vi "rsscope_core_global.vi"() -> ()   [LabVIEW 2014] (continued)
of the data signal in the USB 3.1 protocol.\n\nAvailable Repeated Capabilities:\nSerialBus: SB1, SB2, SB3, SB4\r\n\nRemote-control command(s):\nBUS<m>:USBThree:THRHigh"}, {"Level"=3, "Class Only"=FALSE, "Identifier"="RSSCOPE_ATTR_PROTOCOL_USB31_GEN1_SCRAMBLE_MODE", "Descriptive Name"="Protocol USB31 Gen1 Scramble Mode", "Data Type"=0, "Command"="BUS{SerialBus}:USBT:SCRM", "Access"=2, "Range Table"="RsScope_rngUSB31Gen1ScrambleMode", "Read Callback"="", "Write Callback"="", "Supported Models"="", "Instrument Options"="K61", "Flags"=0, "Help"="Selects if the data pattern is scrambled or unscambled.\n\nAvailable Repeated Capabilities:\nSerialBus: SB1, SB2, SB3, SB4\r\n\nRemote-control command(s):\nBUS<m>:USBThree:SCRMode"}, {"Level"=3, "Class Only"=FALSE, "Identifier"="RSSCOPE_ATTR_PROTOCOL_USB31_GEN1_TYPE", "Descriptive Name"="Protocol USB31 Gen1 Type", "Data Type"=0, "Command"="BUS{SerialBus}:USBT:TYPE", "Access"=2, "Range Table"="RsScope_rngProtocolUSB31Gen1Type", "Read Callback"="", "Write Callback"="", "Supported Models"="", "Instrument Options"="K61", "Flags"=0, "Help"="Selects the USB 3.1 protocol type.\n\nAvailable Repeated Capabilities:\nSerialBus: SB1, SB2, SB3, SB4\r\n\nRemote-control command(s):\nBUS<m>:USBThree:TYPE"}, {"Level"=3, "Class Only"=TRUE, "Identifier"="", "Descriptive Name"="Decoding Results", "Data Type"=0, "Command"="", "Access"=0, "Range Table"="", "Read Callback"="", "Write Callback"="", "Supported Models"="", "Instrument Options"="", "Flags"=0, "Help"="Returns the USB31 Generation1 decoding results."}, {"Level"=4, "Class Only"=FALSE, "Identifier"="RSSCOPE_ATTR_PROTOCOL_USB31_GEN1_FRAME_COUNT", "Descriptive Name"="Protocol USB31 Gen1 Frame Count", "Data Type"=0, "Command"="BUS{SerialBus}:USBT:RES:FCO?", "Access"=0, "Range Table"="", "Read Callback"="", "Write Callback"="", "Supported Models"="", "Instrument Options"="K61", "Flags"=0, "Help"="Returns the number of frames in the acquisition.\n\nAvailable Repeated Capabilities:\nSerialBus: SB1, SB2, SB3, SB4\r\n\nRemote-control command(s):\nBUS<m>:USBThree:RESult:FCOunt?"}, {"Level"=3, "Class Only"=TRUE, "Identifier"="", "Descriptive Name"="DSP", "Data Type"=0, "Command"="", "Access"=0, "Range Table"="", "Read Callback"="", "Write Callback"="", "Supported Models"="", "Instrument Options"="", "Flags"=0, "Help"="Here you can enable and define the equalization techniques used for the equalization at the reciever side of the signal."}, {"Level"=4, "Class Only"=FALSE, "Identifier"="RSSCOPE_ATTR_PROTOCOL_USB31_GEN1_TYPE_DSP_HIGH_SPEED_BITRATE", "Descriptive Name"="Protocol USB31 Gen1 Type DSP High Speed Bitrate", "Data Type"=1, "Command"="BUS{SerialBus}:USBT:BITR", "Access"=2, "Range Table"="RsScope_rngProtocolUSB31Gen1TypeDSPHighSpeedBitrate", "Read Callback"="", "Write Callback"="", "Supported Models"="", "Instrument Options"="K61", "Flags"=0, "Help"="Sets the bit rate.\n\nAvailable Repeated Capabilities:\nSerialBus: SB1, SB2, SB3, SB4\r\n\nRemote-control command(s):\nBUS<m>:USBThree:BITR"}, {"Level"=4, "Class Only"=TRUE, "Identifier"="", "Descriptive Name"="CTLE", "Data Type"=0, "Command"="", "Access"=0, "Range Table"="", "Read Callback"="", "Write Callback"="", "Supported Models"="", "Instrument Options"="", "Flags"=0, "Help"="Continuous time linear equalization (CTLE) is an equalization that can be used for improving the signal performance. It boosts the high frequency noise and the signal. Thus it helps reduce the inter-symbol interference (ISI) on the reciever side."}, {"Level"=5, "Class Only"=FALSE, "Identifier"="RSSCOPE_ATTR_PROTOCOL_USB31_GEN1_TYPE_DSP_CTLE_ENABLED", "Descriptive Name"="Protocol USB31 Gen1 Type DSP CTLE Enabled", "Data Type"=3, "Command"="BUS{SerialBus}:CTLE:ENBL", "Access"=2, "Range Table"="", "Read Callback"="", "Write Callback"="", "Supported Models"="", "Instrument Options"="K61", "Flags"=0, "Help"="Enables the continuous time linear equalization (CTLE) equalization.\n\nAvailable Repeated Capabilities:\nSerialBus: SB1, SB2, SB3, SB4\r\n\nRemote-control command(s):\nBUS<m>:CTLE:ENBLe"}, {"Level"=5, "Class Only"=FALSE, "Identifier"="RSSCOPE_ATTR_PROTOCOL_USB31_GEN1_TYPE_DSP_CTLE_ZERO_FREQUENCY", "Descriptive Name"="Protocol USB31 Gen1 Type DSP CTLE Zero Frequency", "Data Type"=1, "Command"="BUS{SerialBus}:CTLE:Z1FR", "Access"=2, "Range Table"="RsScope_rngProtocolUSB31Gen1TypeDSPCTLEFrequency", "Read Callback"="", "Write Callback"="", "Supported Models"="", "Instrument Options"="K61", "Flags"=0, "Help"="Sets the zero frequency for the transfer function of the CTLE algorithm.\n\nAvailable Repeated Capabilities:\nSerialBus: SB1, SB2, SB3, SB4\r\n\nRemote-control command(s):\nBUS<m>:CTLE:Z1FReq"}, {"Level"=5, "Class Only"=FALSE, "Identifier"="RSSCOPE_ATTR_PROTOCOL_USB31_GEN1_TYPE_DSP_CTLE_POLE_FREQUENCY_FP1", "Descriptive Name"="Protocol USB31 Gen1 Type DSP CTLE Pole Frequency FP1", "Data Type"=1, "Command"="BUS{SerialBus}:CTLE:P1FR", "Access"=2, "Range Table"="RsScope_rngProtocolUSB31Gen1TypeDSPCTLEFrequency", "Read Callback"="", "Write Callback"="", "Supported Models"="", "Instrument Options"="K61", "Flags"=0, "Help"="Sets the pole 1 frequency for the transfer function of the CTLE algorithm.\n\nAvailable Repeated Capabilities:\nSerialBus: SB1, SB2, SB3, SB4\r\n\nRemote-control command(s):\nBUS<m>:CTLE:P1FReq"}, {"Level"=5, "Class Only"=FALSE, "Identifier"="RSSCOPE_ATTR_PROTOCOL_USB31_GEN1_TYPE_DSP_CTLE_POLE_FREQUENCY_FP2", "Descriptive Name"="Protocol USB31 Gen1 Type DSP CTLE Pole Frequency FP2", "Data Type"=1, "Command"="BUS{SerialBus}:CTLE:P2FR", "Access"=2, "Range Table"="RsScope_rngProtocolUSB31Gen1TypeDSPCTLEFrequency", "Read Callback"="", "Write Callback"="", "Supported Models"="", "Instrument Options"="K61", "Flags"=0, "Help"="Sets the pole 2 frequency for the transfer function of the CTLE algorithm.\n\nAvailable Repeated Capabilities:\nSerialBus: SB1, SB2, SB3, SB4\r\n\nRemote-control command(s):\nBUS<m>:CTLE:P2FReq"}, {"Level"=5, "Class Only"=FALSE, "Identifier"="RSSCOPE_ATTR_PROTOCOL_USB31_GEN1_TYPE_DSP_CTLE_DC_GAIN", "Descriptive Name"="Protocol USB31 Gen1 Type DSP CTLE DC Gain", "Data Type"=1, "Command"="BUS{SerialBus}:CTLE:DCG", "Access"=2, "Range Table"="RsScope_rngProtocolUSB31Gen1TypeDSPCTLEDCGain", "Read Callback"="", "Write Callback"="", "Supported Models"="", "Instrument Options"="K61", "Flags"=0, "Help"="Sets the adjustable DC gain. This value can be chosen according to the channel loss characteristics. For low-loss channels, you can set a value close to 0 dB.\n\nAvailable Repeated Capabilities:\nSerialBus: SB1, SB2, SB3, SB4\r\n\nRemote-control command(s):\nBUS<m>:CTLE:DCGain"}, {"Level"=5, "Class Only"=FALSE, "Identifier"="RSSCOPE_ATTR_PROTOCOL_USB31_GEN1_TYPE_DSP_CTLE_CHANNEL_LENGTH", "Descriptive Name"="Protocol USB31 Gen1 Type DSP CTLE Channel Length", "Data Type"=0, "Command"="BUS{SerialBus}:USBT:PROT", "Access"=2, "Range Table"="RsScope_rngUSBDSPChannelLength", "Read Callback"="", "Write Callback"="", "Supported Models"="", "Instrument Options"="K61", "Flags"=0, "Help"="Selects the USB Super Speed channel length.\n\nAvailable Repeated Capabilities:\nSerialBus: SB1, SB2, SB3, SB4\r\n\nRemote-control command(s):\nBUS<m>:USBThree:PROTocol"}, {"Level"=4, "Class Only"=TRUE, "Identifier"="", "Descriptive Name"="DFE", "Data Type"=0, "Command"="", "Access"=0, "Range Table"="", "Read Callback"="", "Write Callback"="", "Supported Models"="", "Instrument Options"="", "Flags"=0, "Help"="Defines the settings of the decision feedback equalization (DFE). DFE correction is needed when the channel is distosrted."}, {"Level"=5, "Class Only"=FALSE, "Identifier"="RSSCOPE_ATTR_PROTOCOL_USB31_GEN1_TYPE_DSP_DFE_ENABLED", "Descriptive Name"="Protocol USB31 Gen1 Type DSP DFE Enabled", "Data Type"=3, "Command"="BUS{SerialBus}:USBT:DFE:ENBL", "Access"=2, "Range Table"="", "Read Callback"="", "Write Callback"="", "Supported Models"="", "Instrument Options"="K61", "Flags"=0, "Help"="Enables the use of the decision feedback equalization for USB 3.1.\n\nAvailable Repeated Capabilities:\nSerialBus: SB1, SB2, SB3, SB4\r\n\nRemote-control command(s):\nBUS<m>:USBThree:DFE:ENBLe"}, {"Level"=5, "Class Only"=FALSE, "Identifier"="RSSCOPE_ATTR_PROTOCOL_USB31_GEN1_TYPE_DSP_DFE_ESTIMATE_COEFFICIENTS_ENABLED", "Descriptive Name"="Protocol USB31 Gen1 Type DSP DFE Estimate Coefficients Enabled", "Data Type"=3, "Command"="BUS{SerialBus}:USBT:DFE:ESTC", "Access"=2, "Range Table"="", "Read Callback"="", "Write Callback"="", "Supported Models"="", "Instrument Options"="K61", "Flags"=0, "Help"="Enables the use of estimate coefficients for the decision feedback equalization.\n\nAvailable Repeated Capabilities:\nSerialBus: SB1, SB2, SB3, SB4\r\n\nRemote-control command(s):\nBUS<m>:USBThree:DFE:ESTCoeff"}, {"Level"=5, "Class Only"=FALSE, "Identifier"="RSSCOPE_ATTR_PROTOCOL_USB31_GEN1_TYPE_DSP_DFE_COEFFICIENT", "Descriptive Name"="Protocol USB31 Gen1 Type DSP DFE Coefficient", "Data Type"=1, "Command"="BUS{SerialBus}:USBT:DFE:COEF", "Access"=2, "Range Table"="RsScope_rngDSPDFECoefficient", "Read Callback"="", "Write Callback"="", "Supported Models"="", "Instrument Options"="K61", "Flags"=0, "Help"="Sets the value of the coefficient for the DFE.\n\nAvailable Repeated Capabilities:\nSerialBus: SB1, SB2, SB3, SB4\r\n\nRemote-control command(s):\nBUS<m>:USBThree:DFE:COEFficient"}, {"Level"=5, "Class Only"=FALSE, "Identifier"="RSSCOPE_ATTR_PROTOCOL_USB31_GEN1_TYPE_DSP_DFE_NUMBER_OF_TAPS", "Descriptive Name"="Protocol USB31 Gen1 Type DSP DFE Number Of Taps", "Data Type"=0, "Command"="BUS{SerialBus}:USBT:DFE:TCON", "Access"=2, "Range Table"="RsScope_rngDSPDFENumberOfTaps", "Read Callback"="", "Write Callback"="", "Supported Models"="", "Instrument Options"="K61", "Flags"=0, "Help"="Sets a number of taps for the decision feedback filter.\n\nAvailable Repeated Capabilities:\nSerialBus: SB1, SB2, SB3, SB4\r\n\nRemote-control command(s):\nBUS<m>:USBThree:DFE:TCONt"}, {"Level"=2, "Class Only"=TRUE, "Identifier"="", "Descriptive Name"="USB PD", "Data Type"=0, "Command"="", "Access"=0, "Range Table"="", "Read Callback"="", "Write Callback"="", "Supported Models"="", "Instrument Options"="", "Flags"=0, "Help"="R&S RTO-K63 is a firmware option that enables the R&S RTO to analyze Universal Serial Bus Power Delivery (USBPD) signals."}, {"Level"=3, "Class Only"=FALSE, "Identifier"="RSSCOPE_ATTR_PROTOCOL_USB_PD_DATA_SOURCE", "Descriptive Name"="Protocol USB PD Data Source", "Data Type"=0, "Command"="BUS{SerialBus}:USBP:SOUR", "Access"=2, "Range Table"="rsscope_rngProtocolWaveformSource", "Read Callback"="", "Write Callback"="", "Supported Models"="", "Instrument Options"="", "Flags"=0, "Help"="Selects the source for the data signal in the USBPD protocol.\n\nAvailable Repeated Capabilities:\nSerialBus: SB1, SB2, SB3, SB4\r\n\nRemote-control command(s):\nBUS<m>:USBPd:SOURce"}, {"Level"=3, "Class Only"=FALSE, "Identifier"="RSSCOPE_ATTR_PROTOCOL_USB_PD_DATA_THRESHOLD", "Descriptive Name"="Protocol USB PD Data Threshold", "Data Type"=1, "Command"="BUS{SerialBus}:USBP:THR", "Access"=2, "Range Table"="RsScope_rngUSBPDThreshold", "Read Callback"="", "Write Callback"="", "Supported Models"="", "Instrument Options"="K63", "Flags"=0, "Help"="Sets the threshold value of the data.\n\nAvailable Repeated Capabilities:\nSerialBus: SB1, SB2, SB3, SB4\r\n\nRemote-control command(s):\nBUS<m>:USBPd:THReshold"}, {"Level"=3, "Class Only"=FALSE, "Identifier"="RSSCOPE_ATTR_PROTOCOL_USB_PD_DATA_HYSTERESIS", "Descriptive Name"="Protocol USB PD Data Hysteresis", "Data Type"=1, "Command"="BUS{SerialBus}:USBP:HYST", "Access"=2, "Range Table"="RsScope_rngUSBPDDataHysteresis", "Read Callback"="", "Write Callback"="", "Supported Models"="", "Instrument Options"="K63", "Flags"=0, "Help"="Sets a value for the hysteresis of the data.\n\nAvailable Repeated Capabilities:\nSerialBus: SB1, SB2, SB3, SB4\r\n\nRemote-control command(s):\nBUS<m>:USBPd:HYSTeresis"}, {"Level"=3, "Class Only"=FALSE, "Identifier"="RSSCOPE_ATTR_PROTOCOL_USB_PD_THRESHOLD_VRD15", "Descriptive Name"="Protocol USB PD Threshold VRD15", "Data Type"=1, "Command"="BUS{SerialBus}:USBP:THRB", "Access"=2, "Range Table"="RsScope_rngUSBPDThreshold", "Read Callback"="", "Write Callback"="", "Supported Models"="", "Instrument Options"="K63", "Flags"=0, "Help"="Sets the bottom threshold (for the low current ) for the current advertisment mode.\n\nAvailable Repeated Capabilities:\nSerialBus: SB1, SB2, SB3, SB4\r\n\nRemote-control command(s):\nBUS<m>:USBPd:THRBottom"}, {"Level"=3, "Class Only"=FALSE, "Identifier"="RSSCOPE_ATTR_PROTOCOL_USB_PD_THRESHOLD_VRD_USB", "Descriptive Name"="Protocol USB PD Threshold VRD USB", "Data Type"=1, "Command"="BUS{SerialBus}:USBP:THRM", "Access"=2, "Range Table"="RsScope_rngUSBPDThreshold", "Read Callback"="", "Write Callback"="", "Supported Models"="", "Instrument Options"="K63", "Flags"=0, "Help"="Sets the middle threshold (at default USB Type-C currnet) for the current advertisment mode.\n\nAvailable Repeated Capabilities:\nSerialBus: SB1, SB2, SB3, SB4\r\n\nRemote-control command(s):\nBUS<m>:USBPd:THRMid"}, {"Level"=3, "Class Only"=FALSE, "Identifier"="RSSCOPE_ATTR_PROTOCOL_USB_PD_THRESHOLD_VRA", "Descriptive Name"="Protocol USB PD Threshold VRA", "Data Type"=1, "Command"="BUS{SerialBus}:USBP:THRT", "Access"=2, "Range Table"="RsScope_rngUSBPDThreshold", "Read Callback"="", "Write Callback"="", "Supported Models"="", "Instrument Options"="K63", "Flags"=0, "Help"="Sets the top threshold (at USB Type-C currnet of 1.5 A ) for the current advertisment mode\n\nAvailable Repeated Capabilities:\nSerialBus: SB1, SB2, SB3, SB4\r\n\nRemote-control command(s):\nBUS<m>:USBPd:THRTop"}, {"Level"=3, "Class Only"=FALSE, "Identifier"="RSSCOPE_ATTR_PROTOCOL_USB_PD_SHOW_DECODE_DETAIL", "Descriptive Name"="Protocol USB PD Show Decode Detail", "Data Type"=3, "Command"="BUS{SerialBus}:USBP:DET", "Access"=2, "Range Table"="", "Read Callback"="", "Write Callback"="", "Supported Models"="", "Instrument Options"="K63", "Flags"=0, "Help"="If enabled, the data words are broken down into subframes. If not enabled the data words are displayed as 32-bit data words.\n\nAvailable Repeated Capabilities:\nSerialBus: SB1, SB2, SB3, SB4\r\n\nRemote-control command(s):\nBUS<m>:USBPd:DETail"}, {"Level"=3, "Class Only"=TRUE, "Identifier"="", "Descriptive Name"="Decoding Results", "Data Type"=0, "Command"="", "Access"=0, "Range Table"="", "Read Callback"="", "Write Callback"="", "Supported Models"="", "Instrument Options"="", "Flags"=0, "Help"="Returns the USB PD decoding results."}, {"Level"=4, "Class Only"=FALSE, "Identifier"="RSSCOPE_ATTR_PROTOCOL_USB_PD_FRAME_COUNT", "Descriptive Name"="Protocol USB PD Frame Count", "Data Type"=0, "Command"="BUS{SerialBus}:USBP:RES:FCO?", "Access"=0, "Range Table"="", "Read Callback"="", "Write Callback"="", "Supported Models"="", "Instrument Options"="K63", "Flags"=0, "Help"="Returns the number of frames in the acquisition.\n\nAvailable Repeated Capabilities:\nSerialBus: SB1, SB2, SB3, SB4\r\n\nRemote-control command(s):\nBUS<m>:USBPd:RESult:FCOunt?"}, {"Level"=2, "Class Only"=TRUE, "Identifier"="", "Descriptive Name"="Custom Manchester NRZ", "Data Type"=0, "Command"="", "Access"=0, "Range Table"="", "Read Callback"="", "Write Callback"="", "Supported Models"="", "Instrument Options"="", "Flags"=0, "Help"="R&S RTO-K50 is a firmware option that enables the R&S RTO to analyze customizable serial bus signals encoded by the following coding standards: Manchester, Manchester II, NRZ Clocked, NRZ Unclocked."}, {"Level"=3, "Class Only"=FALSE, "Identifier"="RSSCOPE_ATTR_PROTOCOL_MANCHESTER_NRZ_CODING_STANDARD", "Descriptive Name"="Protocol Manchester NRZ Coding Standard", "Data Type"=0, "Command"="BUS{SerialBus}:CMSB:COD", "Access"=2, "Range Table"="RsScope_rngManchesterNRZCodingStandard", "Read Callback"="", "Write Callback"="", "Supported Models"="", "Instrument Options"="K50", "Flags"=0, "Help"="Selects the custom serial bus coding standard.\n\nAvailable Repeated Capabilities:\nSerialBus: SB1, SB2, SB3, SB4\r\n\nRemote-control command(s):\nBUS<m>:CMSB:CODing"}, {"Level"=3, "Class Only"=FALSE, "Identifier"="RSSCOPE_ATTR_PROTOCOL_MANCHESTER_NRZ_BITRATE_ENABLED", "Descriptive Name"="Protocol Manchester NRZ Bitrate Enabled", "Data Type"=3, "Command"="BUS{SerialBus}:CMSB:BITR:ENAB", "Access"=2, "Range Table"="", "Read Callback"="", "Write Callback"="", "Supported Models"="", "Instrument Options"="K50", "Flags"=0, "Help"="Enables the bit rate settings (must always be enabled for the coding standard &apos;NRZ Unclocked&apos;, and also for triggering on signals in any coding standard).\n\nAvailable Repeated Capabilities:\nSerialBus: SB1, SB2, SB3, SB4\r\n\nRemote-control command(s):\nBUS<m>:CMSB:BITRate:ENABle"}, {"Level"=3, "Class Only"=FALSE, "Identifier"="RSSCOPE_ATTR_PROTOCOL_MANCHESTER_NRZ_BITRATE", "Descriptive Name"="Protocol Manchester NRZ Bitrate", "Data Type"=0, "Command"="BUS{SerialBus}:CMSB:BITR:VAL", "Access"=2, "Range Table"="RsScope_rngManchesterNRZBitrate", "Read Callback"="", "Write Callback"="", "Supported Models"="", "Instrument Options"="K50", "Flags"=0, "Help"="Sets the transmission speed setting for the custom serial bus data signal.\n\nAvailable Repeated Capabilities:\nSerialBus: SB1, SB2, SB3, SB4\r\n\nRemote-control command(s):\nBUS<m>:CMSB:BITRate:VALue"}, {"Level"=3, "Class Only"=FALSE, "Identifier"="RSSCOPE_ATTR_PROTOCOL_MANCHESTER_NRZ_GAP_TIME_ENABLED", "Descriptive Name"="Protocol Manchester NRZ Gap Time Enabled", "Data Type"=3, "Command"="BUS{SerialBus}:CMSB:GAPT:ENAB", "Access"=2, "Range Table"="", "Read Callback"="", "Write Callback"="", "Supported Models"="", "Instrument Options"="K50", "Flags"=0, "Help"="Enables the gap time settings (must always be enabled for the coding standard &apos;NRZ Unclocked&apos;, and also for triggering on signals in any coding standard).\n\nAvailable Repeated Capabilities:\nSerialBus: SB1, SB2, SB3, SB4\r\n\nRemote-control command(s):\nBUS<m>:CMSB:GAPTime:ENABle"}, {"Level"=3, "Class Only"=FALSE, "Identifier"="RSSCOPE_ATTR_PROTOCOL_MANCHESTER_NRZ_GAP_TIME", "Descriptive Name"="Protocol Manchester NRZ Gap Time", "Data Type"=1, "Command"="BUS{SerialBus}:CMSB:GAPT:VAL", "Access"=2, "Range Table"="RsScope_rngManchesterNRZGapTime", "Read Callback"="", "Write Callback"="", "Supported Models"="", "Instrument Options"="K50", "Flags"=0, "Help"="Sets a minimum gap time for synchronization.\n\nAvailable Repeated Capabilities:\nSerialBus: SB1, SB2, SB3, SB4\r\n\nRemote-control command(s):\nBUS<m>:CMSB:GAPTime:VALue"}, {"Level"=3, "Class Only"=TRUE, "Identifier"="", "Descriptive Name"="Manchester", "Data Type"=0, "Command"="", "Access"=0, "Range Table"="", "Read Callback"="", "Write Callback"="", "Supported Models"="", "Instrument Options"="", "Flags"=0, "Help"="Configures manchester coding standard."}, {"Level"=4, "Class Only"=FALSE, "Identifier"="RSSCOPE_ATTR_PROTOCOL_MANCHESTER_DATA_SOURCE", "Descriptive Name"="Protocol Manchester Data Source", "Data Type"=0, "Command"="BUS{SerialBus}:CMSB:MANC:DATA", "Access"=2, "Range Table"="rsscope_rngProtocolWaveformSource", "Read Callback"="", "Write Callback"="", "Supported Models"="", "Instrument Options"="K50", "Flags"=0, "Help"="Selects the source channel for the data signal. For triggering on a serial bus, analog channels C1 - C4  are required. Otherwise, if no serial bus trigger has been selected, permitted source selections include the mathematical channels and the reference channels.\n\nAvailable Repeated Capabilities:\nSerialBus: SB1, SB2, SB3, SB4\r\n\nRemote-control command(s):\nBUS<m>:CMSB:MANChester:DATA"}, {"Level"=4, "Class Only"=FALSE, "Identifier"="RSSCOPE_ATTR_PROTOCOL_MANCHESTER_POLARITY", "Descriptive Name"="Protocol Manchester Polarity", "Data Type"=0, "Command"="BUS{SerialBus}:CMSB:MANC:POL", "Access"=2, "Range Table"="rsscope_rngPolarityNormalInverted", "Read Callback"="", "Write Callback"="", "Supported Models"="", "Instrument Options"="K50", "Flags"=0, "Help"="Selects the polarity of the custom serial bus data signal in Manchester coding standards.\n\nAvailable Repeated Capabilities:\nSerialBus: SB1, SB2, SB3, SB4\r\n\nRemote-control command(s):\nBUS<m>:CMSB:MANChester:POLarity"}, {"Level"=4, "Class Only"=FALSE, "Identifier"="RSSCOPE_ATTR_PROTOCOL_MANCHESTER_CLOCK_PHASE", "Descriptive Name"="Protocol Manchester Clock Phase", "Data Type"=0, "Command"="BUS{SerialBus}:CMSB:MANC:CPH", "Access"=2, "Range Table"="RsScope_rngClockPhase", "Read Callback"="", "Write Callback"="", "Supported Models"="", "Instrument Options"="K50", "Flags"=0, "Help"="Selects the phase of the custom serial bus clock signal for the &apos;Manchester&apos; coding standards.\n\nAvailable Repeated Capabilities:\nSerialBus: SB1, SB2, SB3, SB4\r\n\nRemote-control command(s):\nBUS<m>:CMSB:MANChester:CPHase"}, {"Level"=4, "Class Only"=FALSE, "Identifier"="RSSCOPE_ATTR_PROTOCOL_MANCHESTER_THRESHOLD_LOW", "Descriptive Name"="Protocol Manchester Threshold Low", "Data Type"=1, "Command"="BUS{SerialBus}:CMSB:MANC:THR:LOW", "Access"=2, "Range Table"="RsScope_rngNRZThreshold", "Read Callback"="", "Write Callback"="", "Supported Models"="", "Instrument Options"="K50", "Flags"=0, "Help"="Sets the lower threshold for data signal digitization in Manchester coding standards.\n\nAvailable Repeated Capabilities:\nSerialBus: SB1, SB2, SB3, SB4\r\n\nRemote-control command(s):\nBUS<m>:CMSB:MANChester:THReshold:LOW"}, {"Level"=4, "Class Only"=FALSE, "Identifier"="RSSCOPE_ATTR_PROTOCOL_MANCHESTER_THRESHOLD_HIGH", "Descriptive Name"="Protocol Manchester Threshold High", "Data Type"=1, "Command"="BUS{SerialBus}:CMSB:MANC:THR:HIGH", "Access"=2, "Range Table"="RsScope_rngProtocolManchesterThresholdHigh", "Read Callback"="", "Write Callback"="", "Supported Models"="", "Instrument Options"="K50", "Flags"=0, "Help"="Sets the upper threshold for data signal digitization in Manchester coding standards.\n\nAvailable Repeated Capabilities:\nSerialBus: SB1, SB2, SB3, SB4\r\n\nRemote-control command(s):\nBUS<m>:CMSB:MANChester:THReshold:HIGH"}, {"Level"=4, "Class Only"=FALSE, "Identifier"="RSSCOPE_ATTR_PROTOCOL_MANCHESTER_THRESHOLD_PRESET", "Descriptive Name"="Protocol Manchester Threshold Preset", "Data Type"=0, "Command"="BUS{SerialBus}:CMSB:MANC:THR:PRES", "Access"=2, "Range Table"="RsScope_rngManchesterNRZThresholdPreset", "Read Callback"="", "Write Callback"="", "Supported Models"="", "Instrument Options"="K50", "Flags"=0, "Help"="Sets the Manchester thresholds to predefined or individually definable voltage levels.\n\nAvailable Repeated Capabilities:\nSerialBus: SB1, SB2, SB3, SB4\r\n\nRemote-control command(s):\nBUS<m>:CMSB:MANChester:THReshold:PRESet"}, {"Level"=4, "Class Only"=FALSE, "Identifier"="RSSCOPE_ATTR_PROTOCOL_MANCHESTER_THRESHOLD_COUPLING", "Descriptive Name"="Protocol Manchester Threshold Coupling", "Data Type"=3, "Command"="BUS{SerialBus}:CMSB:MANC:THR:COUP", "Access"=2, "Range Table"="", "Read Callback"="", "Write Callback"="", "Supported Models"="", "Instrument Options"="K50", "Flags"=0, "Help"="Couples the upper and lower threshold values for the Manchester and Manchester II coding standards. The values are coupled to voltages with the same magnitude but opposite sign (positive for the upper threshold and negative for the lower threshold).\n\nAvailable Repeated Capabilities:\nSerialBus: SB1, SB2, SB3, SB4\r\n\nRemote-control command(s):\nBUS<m>:CMSB:MANChester:THReshold:COUPling"}, {"Level"=3, "Class Only"=TRUE, "Identifier"="", "Descriptive Name"="NRZ", "Data Type"=0, "Command"="", "Access"=0, "Range Table"="", "Read Callback"="", "Write Callback"="", "Supported Models"="", "Instrument Options"="", "Flags"=0, "Help"="Configures NRZ coding standard."}, {"Level"=4, "Class Only"=FALSE, "Identifier"="RSSCOPE_ATTR_PROTOCOL_NRZ_DATA_SOURCE", "Descriptive Name"="Protocol NRZ Data Source", "Data Type"=0, "Command"="BUS{SerialBus}:CMSB:NRZ:DATA", "Access"=2, "Range Table"="rsscope_rngProtocolWaveformSource", "Read Callback"="", "Write Callback"="", "Supported Models"="", "Instrument Options"="K50", "Flags"=0, "Help"="Selects the source channel for the data signal in NRZ coding standards. For triggering on the serial bus when the NRZ clocked coding standard is selected, analog or digital channel sources are required. For triggering on the serial bus when the NRZ unclocked coding standard is selected, analog channel sources are required. Otherwise, if no serial bus trigger has been selected, permitted source selections include the mathematical channels and the reference channels.\n\nAvailable Repeated Capabilities:\nSerialBus: SB1, SB2, SB3, SB4\r\n\nRemote-control command(s):\nBUS<m>:CMSB:NRZ:DATA"}, {"Level"=4, "Class Only"=FALSE, "Identifier"="RSSCOPE_ATTR_PROTOCOL_NRZ_ENABLE_SOURCE", "Descriptive Name"="Protocol NRZ Enable Source", "Data Type"=0, "Command"="BUS{SerialBus}:CMSB:NRZ:ENBL", "Access"=2, "Range Table"="rsscope_rngProtocolWaveformSource", "Read Callback"="", "Write Callback"="", "Supported Models"="", "Instrument Options"="K50", "Flags"=0, "Help"="Selects the input source for the custom serial bus enable signal.\nIf an input is chosen, signals will be only decoded while this channel is in the enabled state. This allows you to mark a time when the signal on the selected source is active and when not.\n\nAvailable Repeated Capabilities:\nSerialBus: SB1, SB2, SB3, SB4\r\n\nRemote-control command(s):\nBUS<m>:CMSB:NRZ:ENBLe"}, {"Level"=4, "Class Only"=FALSE, "Identifier"="RSSCOPE_ATTR_PROTOCOL_NRZ_CLOCK_SOURCE", "Descriptive Name"="Protocol NRZ Clock Source", "Data Type"=0, "Command"="BUS{SerialBus}:CMSB:NRZ:CLCK", "Access"=2, "Range Table"="rsscope_rngProtocolWaveformSource", "Read Callback"="", "Write Callback"="", "Supported Models"="", "Instrument Options"="K50", "Flags"=0, "Help"="Selects the source channel for the clock signal in the NRZ Clocked coding standard. For triggering on the serial bus when the NRZ clocked coding standard is selected, analog or digital channel sources are required. Otherwise, if no serial bus trigger has been selected, permitted source selections include the mathematical channels and the reference channels.\n\nAvailable Repeated Capabilities:\nSerialBus: SB1, SB2, SB3, SB4\r\n\nRemote-control command(s):\nBUS<m>:CMSB:NRZ:CLCK"}, {"Level"=4, "Class Only"=FALSE, "Identifier"="RSSCOPE_ATTR_PROTOCOL_NRZ_POLARITY", "Descriptive Name"="Protocol NRZ Polarity", "Data Type"=0, "Command"="BUS{SerialBus}:CMSB:NRZ:POL", "Access"=2, "Range Table"="rsscope_rngActivePolarity", "Read Callback"="", "Write Callback"="", "Supported Models"="", "Instrument Options"="K50", "Flags"=0, "Help"="Selects the polarity of the custom serial bus data signal in NRZ coding standards.\n\nAvailable Repeated Capabilities:\nSerialBus: SB1, SB2, SB3, SB4\r\n\nRemote-control command(s):\nBUS<m>:CMSB:NRZ:POLarity"}, {"Level"=4, "Class Only"=FALSE, "Identifier"="RSSCOPE_ATTR_PROTOCOL_NRZ_ENA_POLARITY", "Descriptive Name"="Protocol NRZ ENA Polarity", "Data Type"=0, "Command"="BUS{SerialBus}:CMSB:NRZ:ENAP", "Access"=2, "Range Table"="RsScope_rngNRZPolarityData", "Read Callback"="", "Write Callback"="", "Supported Models"="", "Instrument Options"="K50", "Flags"=0, "Help"="Sets whether the transmitted enable signal is active when the voltage is below the threshold (ENALow) or higher than it (ENAHIgh).\n\nAvailable Repeated Capabilities:\nSerialBus: SB1, SB2, SB3, SB4\r\n\nRemote-control command(s):\nBUS<m>:CMSB:NRZ:ENAPolarity"}, {"Level"=4, "Class Only"=FALSE, "Identifier"="RSSCOPE_ATTR_PROTOCOL_NRZ_IDLE_POLARITY_UNCLOCKED", "Descriptive Name"="Protocol NRZ Idle Polarity Unclocked", "Data Type"=0, "Command"="BUS{SerialBus}:CMSB:NRZ:IDLP", "Access"=2, "Range Table"="rsscope_rngProtocolPolarity", "Read Callback"="", "Write Callback"="", "Supported Models"="", "Instrument Options"="K50", "Flags"=0, "Help"="Selects the idle polarity of the custom serial bus data signal (only available for the coding standard &apos;NRZ Unclocked&apos;).\n\nAvailable Repeated Capabilities:\nSerialBus: SB1, SB2, SB3, SB4\r\n\nRemote-control command(s):\nBUS<m>:CMSB:NRZ:IDLPolarity"}, {"Level"=4, "Class Only"=FALSE, "Identifier"="RSSCOPE_ATTR_PROTOCOL_NRZ_IDLE_POLARITY_CLOCKED", "Descriptive Name"="Protocol NRZ Idle Polarity Clocked", "Data Type"=0, "Command"="BUS{SerialBus}:CMSB:NRZ:CPOL", "Access"=2, "Range Table"="rsscope_rngProtocolPolarity", "Read Callback"="", "Write Callback"="", "Supported Models"="", "Instrument Options"="K50", "Flags"=0, "Help"="Selects the custom serial bus clock signal polarity for the coding standard NRZ Clocked.\n\nAvailable Repeated Capabilities:\nSerialBus: SB1, SB2, SB3, SB4\r\n\nRemote-control command(s):\nBUS<m>:CMSB:NRZ:CPOLarity"}, {"Level"=4, "Class Only"=FALSE, "Identifier"="RSSCOPE_ATTR_PROTOCOL_NRZ_CLOCK_PHASE", "Descriptive Name"="Protocol NRZ Clock Phase", "Data Type"=0, "Command"="BUS{SerialBus}:CMSB:NRZ:CPH", "Access"=2, "Range Table"="RsScope_rngNRZClockPhase", "Read Callback"="", "Write Callback"="", "Supported Models"="", "Instrument Options"="K50", "Flags"=0, "Help"="Selects the phase of the custom serial bus clock signal for the NRZ coding standards.\n\nAvailable Repeated Capabilities:\nSerialBus: SB1, SB2, SB3, SB4\r\n\nRemote-control command(s):\nBUS<m>:CMSB:NRZ:CPHase"}, {"Level"=4, "Class Only"=FALSE, "Identifier"="RSSCOPE_ATTR_PROTOCOL_NRZ_THRESHOLD_CLOCK", "Descriptive Name"="Protocol NRZ Threshold Clock", "Data Type"=1, "Command"="BUS{SerialBus}:CMSB:NRZ:THR:CLCK", "Access"=2, "Range Table"="RsScope_rngNRZThreshold", "Read Callback"="", "Write Callback"="", "Supported Models"="", "Instrument Options"="K50", "Flags"=0, "Help"="Sets the threshold for the clock signal digitization in the NRZ Clocked coding standard.\n\nAvailable Repeated Capabilities:\nSerialBus: SB1, SB2, SB3, SB4\r\n\nRemote-control command(s):\nBUS<m>:CMSB:NRZ:THReshold:CLCK"}, {"Level"=4, "Class Only"=FALSE, "Identifier"="RSSCOPE_ATTR_PROTOCOL_NRZ_THRESHOLD_DATA", "Descriptive Name"="Protocol NRZ Threshold Data", "Data Type"=1, "Command"="BUS{SerialBus}:CMSB:NRZ:THR:DATA", "Access"=2, "Range Table"="RsScope_rngNRZThreshold", "Read Callback"="", "Write Callback"="", "Supported Models"="", "Instrument Options"="K50", "Flags"=0, "Help"="Sets the threshold for the data signal digitization in NRZ coding standards.\n\nAvailable Repeated Capabilities:\nSerialBus: SB1, SB2, SB3, SB4\r\n\nRemote-control command(s):\nBUS<m>:CMSB:NRZ:THReshold:DATA"}, {"Level"=4, "Class Only"=FALSE, "Identifier"="RSSCOPE_ATTR_PROTOCOL_NRZ_THRESHOLD_PRESET", "Descriptive Name"="Protocol NRZ Threshold Preset", "Data Type"=0, "Command"="BUS{SerialBus}:CMSB:NRZ:THR:PRES", "Access"=2, "Range Table"="RsScope_rngManchesterNRZThresholdPreset", "Read Callback"="", "Write Callback"="", "Supported Models"="", "Instrument Options"="K50", "Flags"=0, "Help"="Sets the NRZ thresholds to predefined or individually definable voltage levels.\n\nAvailable Repeated Capabilities:\nSerialBus: SB1, SB2, SB3, SB4\r\n\nRemote-control command(s):\nBUS<m>:CMSB:NRZ:THReshold:PRESet"}, {"Level"=4, "Class Only"=FALSE, "Identifier"="RSSCOPE_ATTR_PROTOCOL_NRZ_THRESHOLD_COUPLING", "Descriptive Name"="Protocol NRZ Threshold Coupling", "Data Type"=3, "Command"="BUS{SerialBus}:CMSB:NRZ:THR:COUP", "Access"=2, "Range Table"="", "Read Callback"="", "Write Callback"="", "Supported Models"="", "Instrument Options"="K50", "Flags"=0, "Help"="Couples the clock and data threshold values for the NRZ Clocked coding standard. The values are coupled to the same number.\n\nAvailable Repeated Capabilities:\nSerialBus: SB1, SB2, SB3, SB4\r\n\nRemote-control command(s):\nBUS<m>:CMSB:NRZ:THReshold:COUPling"}, {"Level"=4, "Class Only"=FALSE, "Identifier"="RSSCOPE_ATTR_PROTOCOL_NRZ_THRESHOLD_VALUE", "Descriptive Name"="Protocol NRZ Threshold Value", "Data Type"=1, "Command"="BUS{SerialBus}:CMSB:NRZ:THR:ENBL", "Access"=2, "Range Table"="RsScope_rngNRZThresholdEnabled", "Read Callback"="", "Write Callback"="", "Supported Models"="", "Instrument Options"="K50", "Flags"=0, "Help"="Sets the threshold for the enable signal digitization in NRZ coding standards.\n\nAvailable Repeated Capabilities:\nSerialBus: SB1, SB2, SB3, SB4\r\n\nRemote-control command(s):\nBUS<m>:CMSB:NRZ:THReshold:ENBLe"}, {"Level"=4, "Class Only"=FALSE, "Identifier"="RSSCOPE_ATTR_PROTOCOL_NRZ_HYSTERESIS_CLOCK", "Descriptive Name"="Protocol NRZ Hysteresis Clock", "Data Type"=1, "Command"="BUS{SerialBus}:CMSB:NRZ:HYST:CLCK", "Access"=2, "Range Table"="RsScope_rngNRZHysteresis", "Read Callback"="", "Write Callback"="", "Supported Models"="", "Instrument Options"="K50", "Flags"=0, "Help"="Sets the hysteresis size on the clock channel.\n\nAvailable Repeated Capabilities:\nSerialBus: SB1, SB2, SB3, SB4\r\n\nRemote-control command(s):\nBUS<m>:CMSB:NRZ:HYSTeresis:CLCK"}, {"Level"=4, "Class Only"=FALSE, "Identifier"="RSSCOPE_ATTR_PROTOCOL_NRZ_HYSTERESIS_DATA", "Descriptive Name"="Protocol NRZ Hysteresis Data", "Data Type"=1, "Command"="BUS{SerialBus}:CMSB:NRZ:HYST:DATA", "Access"=2, "Range Table"="RsScope_rngNRZHysteresis", "Read Callback"="", "Write Callback"="", "Supported Models"="", "Instrument Options"="K50", "Flags"=0, "Help"="Sets the hysteresis size on the data line channel.\n\nAvailable Repeated Capabilities:\nSerialBus: SB1, SB2, SB3, SB4\r\n\nRemote-control command(s):\nBUS<m>:CMSB:NRZ:HYSTeresis:DATA"}, {"Level"=4, "Class Only"=FALSE, "Identifier"="RSSCOPE_ATTR_PROTOCOL_NRZ_HYSTERESIS_ENABLE_VALUE", "Descriptive Name"="Protocol NRZ Hysteresis Enable Value", "Data Type"=1, "Command"="BUS{SerialBus}:CMSB:NRZ:HYST:ENBL", "Access"=2, "Range Table"="RsScope_rngNRZHysteresis", "Read Callback"="", "Write Callback"="", "Supported Models"="", "Instrument Options"="K50", "Flags"=0, "Help"="Sets the hysteresis size on the enable line channel.\n\nAvailable Repeated Capabilities:\nSerialBus: SB1, SB2, SB3, SB4\r\n\nRemote-control command(s):\nBUS<m>:CMSB:NRZ:HYSTeresis:ENBLe"}, {"Level"=3, "Class Only"=TRUE, "Identifier"="", "Descriptive Name"="Frame Format", "Data Type"=0, "Command"="", "Access"=0, "Range Table"="", "Read Callback"="", "Write Callback"="", "Supported Models"="", "Instrument Options"="", "Flags"=0, "Help"="Configures frame format."}, {"Level"=4, "Class Only"=FALSE, "Identifier"="RSSCOPE_ATTR_PROTOCOL_MANCHESTER_NRZ_SELECTED_FRAME", "Descriptive Name"="Protocol Manchester NRZ Selected Frame", "Data Type"=0, "Command"="", "Access"=2, "Range Table"="", "Read Callback"="", "Write Callback"="", "Supported Models"="", "Instrument Options"="", "Flags"=0, "Help"="Sets selector repeated capability Frame.\n\nAvailable Repeated Capabilities:\nNone\n\nRemote-control command(s):\n"}, {"Level"=4, "Class Only"=FALSE, "Identifier"="RSSCOPE_ATTR_PROTOCOL_MANCHESTER_NRZ_FRAME_COUNT", "Descriptive Name"="Protocol Manchester NRZ Frame Count", "Data Type"=0, "Command"="BUS{SerialBus}:CMSB:FCO?", "Access"=0, "Range Table"="", "Read Callback"="", "Write Callback"="", "Supported Models"="", "Instrument Options"="K50", "Flags"=0, "Help"="Returns the frame count.\n\nAvailable Repeated Capabilities:\nSerialBus: SB1, SB2, SB3, SB4\r\n\nRemote-control command(s):\nBUS<m>:CMSB:FCOunt?"}, {"Level"=4, "Class Only"=FALSE, "Identifier"="RSSCOPE_ATTR_PROTOCOL_MANCHESTER_NRZ_FRAME_TYPE", "Descriptive Name"="Protocol Manchester NRZ Frame Type", "Data Type"=2, "Command"="BUS{SerialBus}:CMSB:FRAM<Frame>:TYPE", "Access"=2, "Range Table"="", "Read Callback"="rsscope_FormatManchesterNRZFrameRepCapString_ReadCallback.vi", "Write Callback"="rsscope_FormatManchesterNRZFrameRepCapString_WriteCallback.vi", "Supported Models"="", "Instrument Options"="K50", "Flags"=0, "Help"="Enables the user to set a string to describe the frame type, typically according to the applicable protocol standard specifications. (For example, MDIO (Option R&S RTO-K55) defines the frames READ, WRITE, ADDRESS, etc.)\n\nAvailable Repeated Capabilities:\nSerialBus: SB1, SB2, SB3, SB4\r\n\nRemote-control command(s):\nBUS<m>:CMSB:FRAMe<n>:TYPE"}, {"Level"=4, "Class Only"=FALSE, "Identifier"="RSSCOPE_ATTR_PROTOCOL_MANCHESTER_NRZ_ADD_FRAME", "Descriptive Name"="Protocol Manchester NRZ Add Frame", "Data Type"=4, "Command"="BUS{SerialBus}:CMSB:ADDF", "Access"=1, "Range Table"="", "Read Callback"="", "Write Callback"="", "Supported Models"="", "Instrument Options"="K50", "Flags"=0, "Help"="Creates an empty frame format description and adds it to the end of the frame description list.\n\nAvailable Repeated Capabilities:\nSerialBus: SB1, SB2, SB3, SB4\r\n\nRemote-control command(s):\nBUS<m>:CMSB:ADDFrame"}, {"Level"=4, "Class Only"=FALSE, "Identifier"="RSSCOPE_ATTR_PROTOCOL_MANCHESTER_NRZ_FRAME_CLEAR", "Descriptive Name"="Protocol Manchester NRZ Frame Clear", "Data Type"=4, "Command"="BUS{SerialBus}:CMSB:CLR", "Access"=1, "Range Table"="", "Read Callback"="", "Write Callback"="", "Supported Models"="", "Instrument Options"="K50", "Flags"=0, "Help"="Erases all cells and frames that have been created for a specific custom protocol.\n\nAvailable Repeated Capabilities:\nSerialBus: SB1, SB2, SB3, SB4\r\n\nRemote-control command(s):\nBUS<m>:CMSB:CLR"}, {"Level"=4, "Class Only"=FALSE, "Identifier"="RSSCOPE_ATTR_PROTOCOL_MANCHESTER_NRZ_FRAME_OPEN_DESCRIPTION", "Descriptive Name"="Protocol Manchester NRZ Frame Open Description", "Data Type"=2, "Command"="BUS{SerialBus}:CMSB:LOAD", "Access"=1, "Range Table"="", "Read Callback"="", "Write Callback"="", "Supported Models"="", "Instrument Options"="K50", "Flags"=0, "Help"="Opens an existing frame description file in xml format. The default path is \\\\Public\\Documents\\Rohde-Schwarz\\RTx\\SaveXML\n\nAvailable Repeated Capabilities:\nSerialBus: SB1, SB2, SB3, SB4\r\n\nRemote-control command(s):\nBUS<m>:CMSB:LOAD"}, {"Level"=4, "Class Only"=FALSE, "Identifier"="RSSCOPE_ATTR_PROTOCOL_MANCHESTER_NRZ_FRAME_SAVE_DESCRIPTION", "Descriptive Name"="Protocol Manchester NRZ Frame Save Description", "Data Type"=2, "Command"="BUS{SerialBus}:CMSB:SAVE", "Access"=1, "Range Table"="", "Read Callback"="", "Write Callback"="", "Supported Models"="", "Instrument Options"="K50", "Flags"=0, "Help"="Saves a created frame description into an xml file (&apos;Save As...&apos;). The default path is \\\\Public\\Documents\\Rohde-Schwarz\\RTx\\SaveXML\n\nAvailable Repeated Capabilities:\nSerialBus: SB1, SB2, SB3, SB4\r\n\nRemote-control command(s):\nBUS<m>:CMSB:SAVE"}, {"Level"=4, "Class Only"=FALSE, "Identifier"="RSSCOPE_ATTR_PROTOCOL_MANCHESTER_NRZ_EXPORT_FRAMES_AS_RAW_BITS", "Descriptive Name"="Protocol Manchester NRZ Export Frames As Raw Bits", "Data Type"=4, "Command"="BUS{SerialBus}:CMSB:EXRB", "Access"=1, "Range Table"="", "Read Callback"="", "Write Callback"="", "Supported Models"="", "Instrument Options"="K50", "Flags"=0, "Help"="Exports the decoded frames as raw bits.\n\nAvailable Repeated Capabilities:\nSerialBus: SB1, SB2, SB3, SB4\r\n\nRemote-control command(s):\nBUS<m>:CMSB:EXRBits"}, {"Level"=4, "Class Only"=TRUE, "Identifier"="", "Descriptive Name"="Cell", "Data Type"=0, "Command"="", "Access"=0, "Range Table"="", "Read Callback"="", "Write Callback"="", "Supported Models"="", "Instrument Options"="", "Flags"=0, "Help"="Configures the cell."}, {"Level"=5, "Class Only"=FALSE, "Identifier"="RSSCOPE_ATTR_PROTOCOL_MANCHESTER_NRZ_SELECTED_CELL", "Descriptive Name"="Protocol Manchester NRZ Selected Cell", "Data Type"=0, "Command"="", "Access"=2, "Range Table"="", "Read Callback"="", "Write Callback"="", "Supported Models"="", "Instrument Options"="", "Flags"=0, "Help"="Sets selector repeated capability Cell.\n\nAvailable Repeated Capabilities:\nNone\n\nRemote-control command(s):\nn"}, {"Level"=5, "Class Only"=FALSE, "Identifier"="RSSCOPE_ATTR_PROTOCOL_MANCHESTER_NRZ_CELL_COUNT", "Descriptive Name"="Protocol Manchester NRZ Cell Count", "Data Type"=0, "Command"="BUS{SerialBus}:CMSB:FRAM<Frame>:CCO?", "Access"=0, "Range Table"="", "Read Callback"="rsscope_FormatManchesterNRZFrameRepCapInt32_ReadCallback.vi", "Write Callback"="rsscope_FormatManchesterNRZFrameRepCapInt32_WriteCallback.vi", "Supported Models"="", "Instrument Options"="K50", "Flags"=0, 
